vi "numCmd_ObtainQueue_TwoDbl.vi"(11 "Command Name":string) -> (0 "error out":errorcluster, 3 "queue out":refnum<queue>)   [LabVIEW 2019, in "Trajectory_Library.lvlib"]
uses:
  Trajectory_Library.lvlib
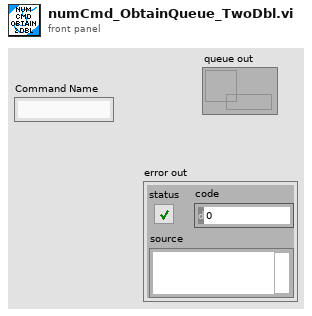
[diagram p1: front panel]
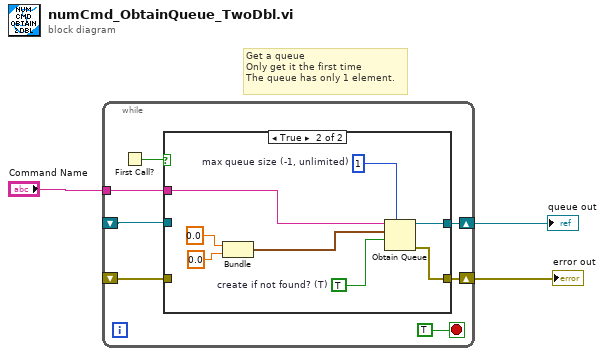
[diagram p0: block diagram]
diagram:
  # "Get a queue\nOnly get it the first time\nThe queue has only 1 element."
  n1 = while {
    tunnel: "Command Name" -> [w10]
    shift-right: [w7] -> w1
    shift-left: _ -> [w6]
    shift-right: [w5] -> w2
    shift-left: _ -> [w4]
    stop <- TRUE stop-if-true
    n2 = First Call?() -> (First Call?: T/F=w8:bool)
    n3 = case shown="True" w8 {
      tunnel: w10 -> [_ w18]
      tunnel: [w12 w17] -> w7
      tunnel: w6 -> [w12 _]
      tunnel: [w11 w16] -> w5
      tunnel: w4 -> [w11 _]
      frame False {
      }
      frame True {
        w19 = TRUE  # create if not found? (T)
        w20 = 1  # max queue size (-1, unlimited)
        n4 = Bundle(0.0, 0.0) -> (w13:cluster{dbl, dbl})  [unwired: 1 in]
        n5 = Obtain Queue(max queue size (-1, unlimited)=w20, name (unnamed)=w18, element data type=w13, create if not found? (T)=w19) -> (queue out=w17:refnum<queue>, error out=w16:errorcluster)  [unwired: 1 in, 1 out]
      }
    }
  }
  "error out" <- w2
  "queue out" <- w1
